vi "CalculateSyncPulse.vi"(11 "VGA_data":T1={"x_frontporch"=0, "x_syncpulse"=0, "x_backporch"=0, "y_frontporch"=0, "y_syncpulse"=0, "y_backporch"=0, "DrawPixel?"=FALSE, "x_tickcount"=0, "y_tickcount"=0, "x_Index"=-1, "y_Index"=-1}) -> (1 "vSync":bool, 2 "hSync":bool, 3 "VGA_data 2":T1={"x_frontporch"=0, "x_syncpulse"=0, "x_backporch"=0, "y_frontporch"=0, "y_syncpulse"=0, "y_backporch"=0, "DrawPixel?"=FALSE, "x_tickcount"=0, "y_tickcount"=0, "x_Index"=-1, "y_Index"=-1})   [LabVIEW 2019, in "VGA.lvlib"]
uses:
  VGA.lvlib
  data.ctl
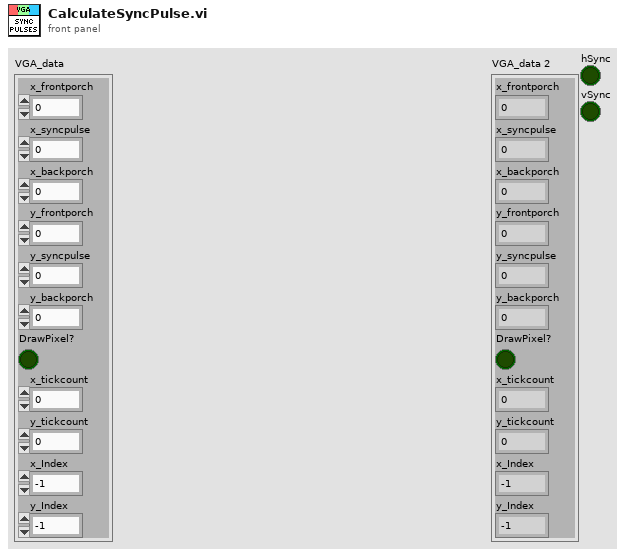
[diagram p1: front panel]
types:
  T1 = typedef "VGA.lvlib/data.ctl" = cluster{"x_frontporch":u8, "x_syncpulse":u8, "x_backporch":u8, "y_frontporch":u8, "y_syncpulse":u8, "y_backporch":u8, "DrawPixel?":bool, "x_tickcount":u16, "y_tickcount":u16, "x_Index":i16, "y_Index":i16}
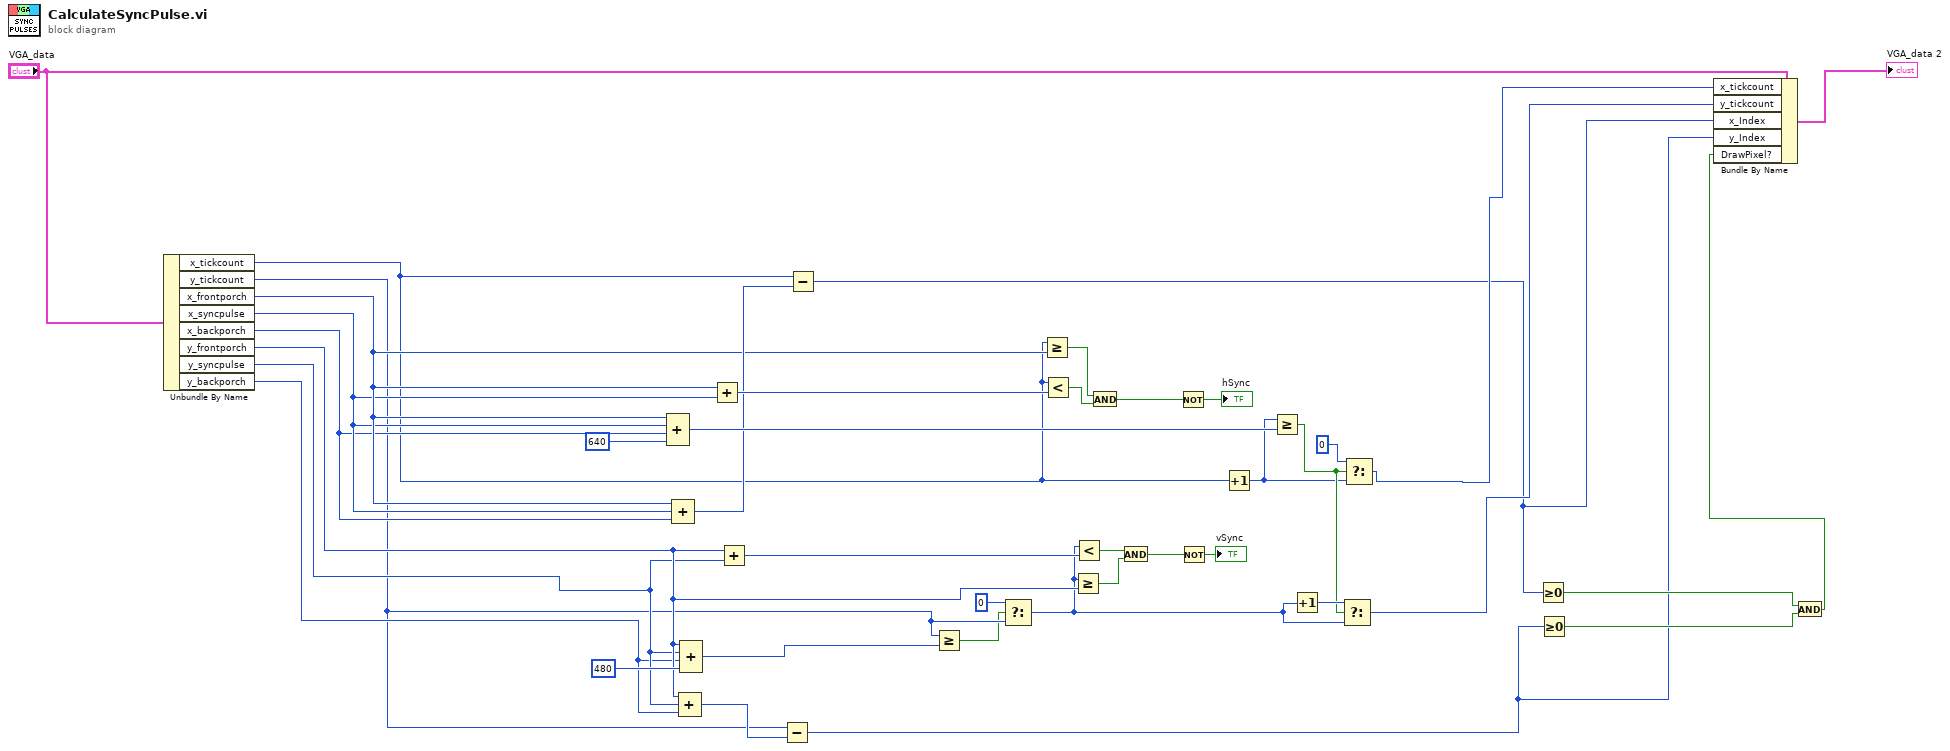
[diagram p0: block diagram]
diagram:
  n1 = Unbundle By Name("VGA_data") -> ("x_tickcount"=w23:u16, "y_tickcount"=w20:u16, "x_frontporch"=w29:u8, "x_syncpulse"=w28:u8, "x_backporch"=w27:u8, "y_frontporch"=w26:u8, "y_syncpulse"=w25:u8, "y_backporch"=w24:u8)
  n2 = Compound Arithmetic op=unknown(w29, w28, w27, u16 640 ("Res_Width (640)")) -> (w36:u16)
  n3 = Compound Arithmetic op=ADD(w29, w28, w27) -> (w33:u8)
  n4 = Compound Arithmetic op=ADD(w26, w25, w24) -> (w32:u8)
  n5 = Compound Arithmetic op=unknown(w26, w25, w24, u16 480 ("Res_Height (480)")) -> (w34:u16)
  n6 = Add(x=w29, y=w28) -> (x+y=w37:u8)
  n7 = Add(x=w26, y=w25) -> (x+y=w35:u8)
  n8 = Subtract(x=w20, y=w32) -> (x-y=w17:i16)
  n9 = Subtract(x=w23, y=w33) -> (x-y=w18:i16)
  n10 = Greater Or Equal?(x=w20, y=w34) -> (x >= y?=w9:bool)
  n11 = Select(t=u16 0, s=w9, f=w20) -> (s? t:f=w13:u16)
  n12 = Greater Or Equal?(x=w23, y=w29) -> (x >= y?=w8:bool)
  n13 = Less?(x=w23, y=w37) -> (x < y?=w7:bool)
  n14 = Greater Or Equal?(x=w13, y=w26) -> (x >= y?=w11:bool)
  n15 = Less?(x=w13, y=w35) -> (x < y?=w12:bool)
  n16 = And(x=w8, y=w7) -> (x .and. y?=w14:bool)
  n17 = And(x=w12, y=w11) -> (x .and. y?=w15:bool)
  n18 = Not(x=w14) -> (.not. x?=→"hSync":bool)
  n19 = Not(x=w15) -> (.not. x?=→"vSync":bool)
  n20 = Increment(x=w23) -> (x+1=w3:u16)
  n21 = Greater Or Equal?(x=w3, y=w36) -> (x >= y?=w5:bool)
  n22 = Increment(x=w13) -> (x+1=w6:u16)
  n23 = Select(t=w6, s=w5, f=w13) -> (s? t:f=w19:u16)
  n24 = Select(t=u16 0, s=w5, f=w3) -> (s? t:f=w21:u16)
  n25 = Greater Or Equal To 0?(x=w18) -> (x >= 0?=w31:bool)
  n26 = Greater Or Equal To 0?(x=w17) -> (x >= 0?=w30:bool)
  n27 = And(x=w31, y=w30) -> (x .and. y?=w16:bool)
  n28 = Bundle By Name(cluster="VGA_data", "x_tickcount"=w21, "y_tickcount"=w19, "x_Index"=w18, "y_Index"=w17, "DrawPixel?"=w16) -> (→"VGA_data 2":T1)
